vi "Read Invert Inputs.vi"(9 "CompoundArithmetic in":refnum<class "CompoundArithmetic.lvclass">) -> (3 "CompoundArithmetic out":refnum<class "CompoundArithmetic.lvclass">, 4 "Invert Inputs":bool[](array[boolean]))   [LabVIEW 2014, in "CompoundArithmetic.lvclass"]
uses:
  CompoundArithmetic.lvclass
  CompoundArithmetic.lvclass/CompoundArithmetic.ctl
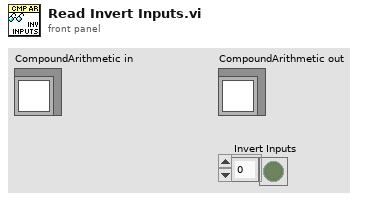
[diagram p1: front panel]
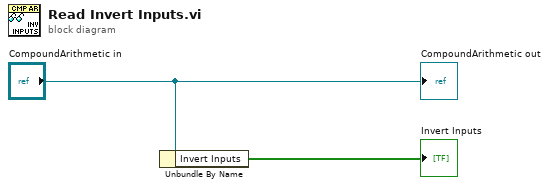
[diagram p0: block diagram]
diagram:
  n1 = Unbundle By Name("CompoundArithmetic in") -> ("Invert Inputs"=→"Invert Inputs":bool[])
  "CompoundArithmetic out" <- "CompoundArithmetic in"
